vi "RingWithKerf.vi"(5 "Center Hole":dbl=1.0 format="%.2f", 6 "kerf?":bool, 7 "kerf space (cm)":dbl format="%.4f", 8 "Trans Geometry":T2={"Radius"=4.8, "a"=1.0, "focus location"=12.0} {"focus location" format="%.2f"; "a" format="%.2f"; "Radius" format="%.2f"}, 9 "Variables":T1={"Number of rings"=1, "sound spd (cm/s)"=150000, "z span (cm)"=4.0, "z steps"=20, "y spacing (cm)"=0.01, "y steps"=50, "time step (s)"=1e-08, "z"=0.0, "y"=0.0, "ref delay"=0.0, "freq (MHz)"=4.71, "cycles"=300} {"freq (MHz)" format="%.2f"; "z span (cm)" format="%.2f"; "y" format="%.2f"; "ref delay" format="%.2f"; "y spacing (cm)" format="%.2f"; "z" format="%.2f"; "time step (s)" format="%.2e"}) -> (0 "refdelay":dbl, 1 "appended array":cluster{"R":dbl, "a":dbl}[][](array[cluster]) {"a" format="%.2f"; "R" format="%.3f"})   [LabVIEW 2022 SP3]
panel:
  in  "Seno 30 mm R 18 mm Ap":cluster{"R":dbl, "a":dbl}[][](array[cluster])=[[{"R"=3.0, "a"=0.25145}, {"R"=0.0, "a"=0.0}], [{"R"=3.0, "a"=0.38285}, {"R"=3.0, "a"=0.28865}], [{"R"=3.0, "a"=0.4896}, {"R"=3.0, "a"=0.42005}], [{"R"=3.0, "a"=0.58375}, {"R"=3.0, "a"=0.5268}], [{"R"=3.0, "a"=0.66995}, {"R"=3.0, "a"=0.62095}], [{"R"=3.0, "a"=0.75055}, {"R"=3.0, "a"=0.70715}], [{"R"=3.0, "a"=0.8269}, {"R"=3.0, "a"=0.78775}], [{"R"=3.0, "a"=0.9}, {"R"=3.0, "a"=0.8641}]]
  in  "Seno 11 mm R 16 mm Ap":cluster{"R":dbl, "a":dbl}[][](array[cluster])=[[{"R"=1.1, "a"=0.2155}, {"R"=0.0, "a"=0.0}], [{"R"=1.1, "a"=0.3322}, {"R"=1.1, "a"=0.2527}], [{"R"=1.1, "a"=0.4277}, {"R"=1.1, "a"=0.3694}], [{"R"=1.1, "a"=0.5124}, {"R"=1.1, "a"=0.4649}], [{"R"=1.1, "a"=0.5904}, {"R"=1.1, "a"=0.5466}], [{"R"=1.1, "a"=0.6636}, {"R"=1.1, "a"=0.6261}], [{"R"=1.1, "a"=0.7332}, {"R"=1.1, "a"=0.7008}], [{"R"=1.1, "a"=0.7999101254524568}, {"R"=1.1, "a"=0.7704}]] {"a" format="%.4f"; "R" format="%.3f"}
  in  "Seno 25 mm R 16 mm App":cluster{"R":dbl, "a":dbl}[][](array[cluster])=[[{"R"=2.5, "a"=0.36477000000000004}, {"R"=0.0, "a"=0.0}], [{"R"=2.5, "a"=0.536}, {"R"=2.5, "a"=0.3972}], [{"R"=2.5, "a"=0.6769}, {"R"=2.5, "a"=0.5732}], [{"R"=2.5, "a"=0.799903752690246}, {"R"=2.5, "a"=0.7141}]] {"a" format="%.3f"; "R" format="%.3f"}
  out "Ring Areas cm^2":dbl[](array[numeric]) format="%.4f"
  # "5.029 \t0.000\n7.657 \t5.773\n9.792 \t8.401\n11.675 \t10.536\n13.399 \t12.419\n15.011 \t14.143\n16.538 \t15.755 \n18.000 \t17.282"
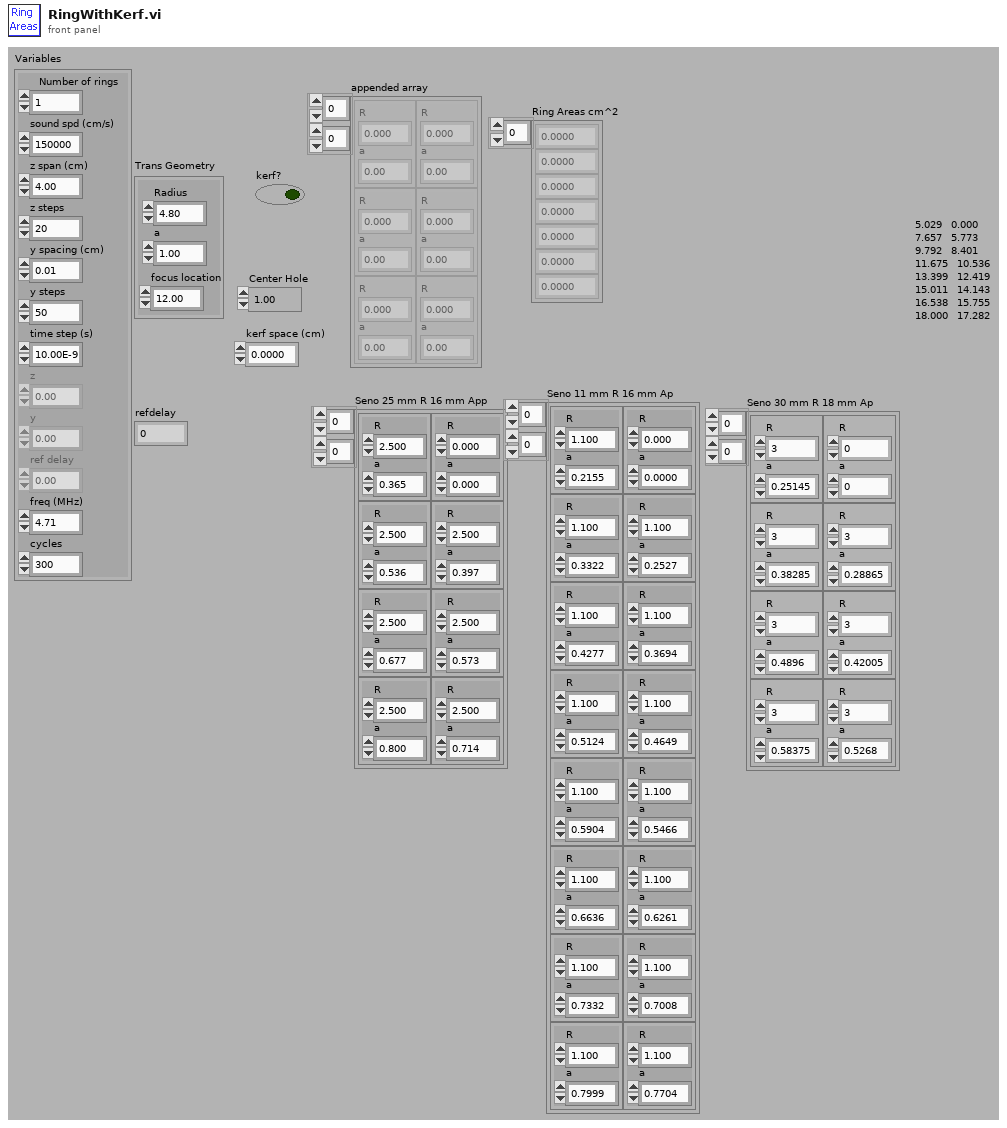
[diagram p1: front panel]
types:
  T1 = cluster{"Number of rings":i32, "sound spd (cm/s)":i32, "z span (cm)":dbl, "z steps":i32, "y spacing (cm)":dbl, "y steps":i32, "time step (s)":sgl, "z":dbl, "y":dbl, "ref delay":dbl, "freq (MHz)":dbl, "cycles":i32}
  T2 = cluster{"Radius":dbl, "a":dbl, "focus location":dbl}
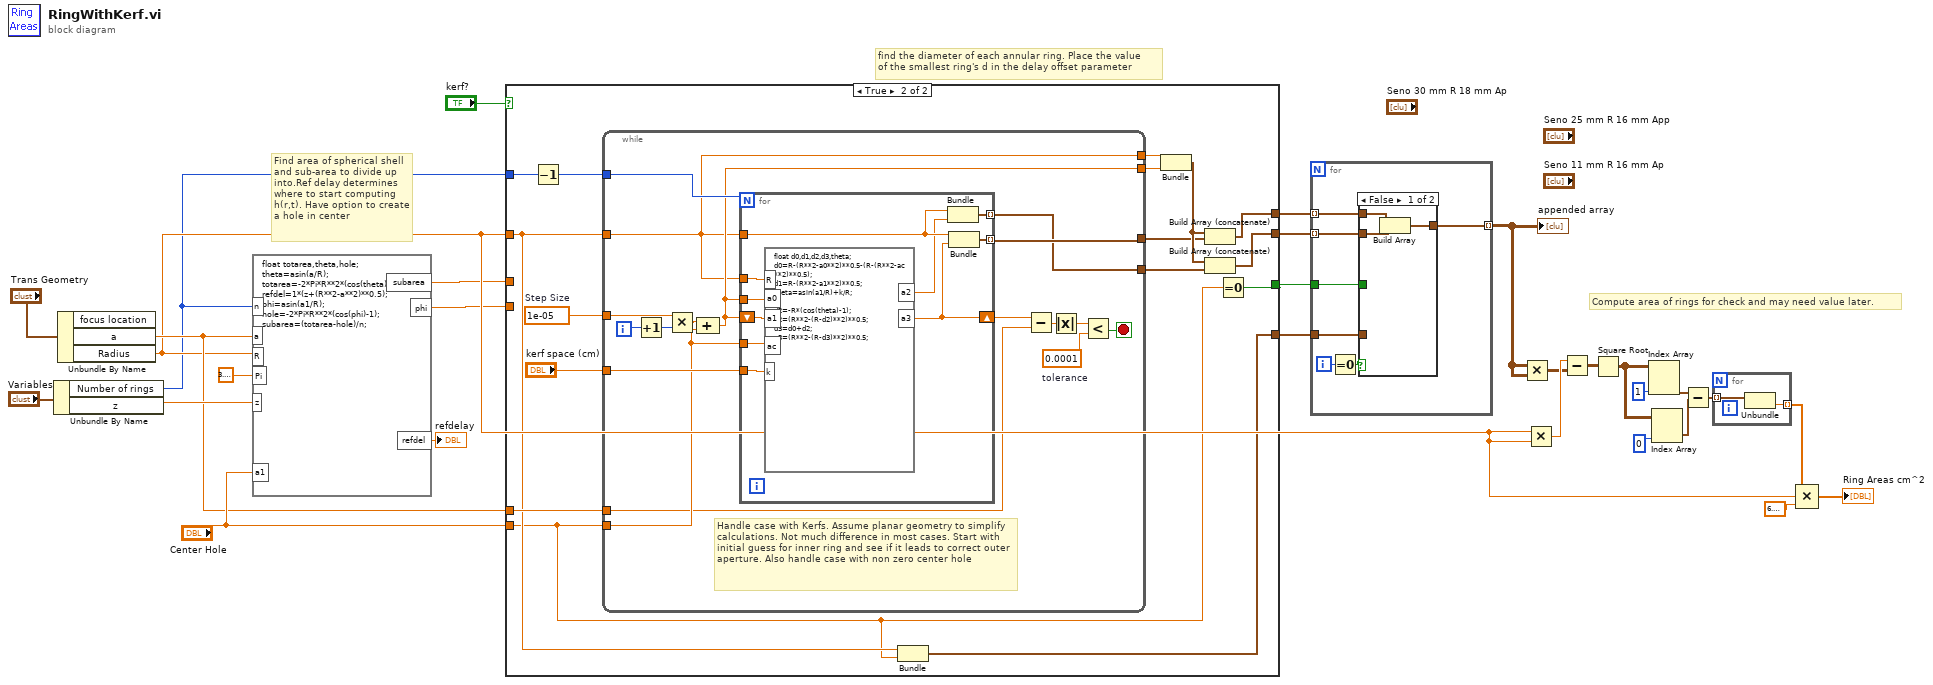
[diagram p0: block diagram]
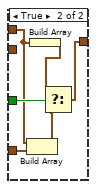
[diagram p2: hidden frame]
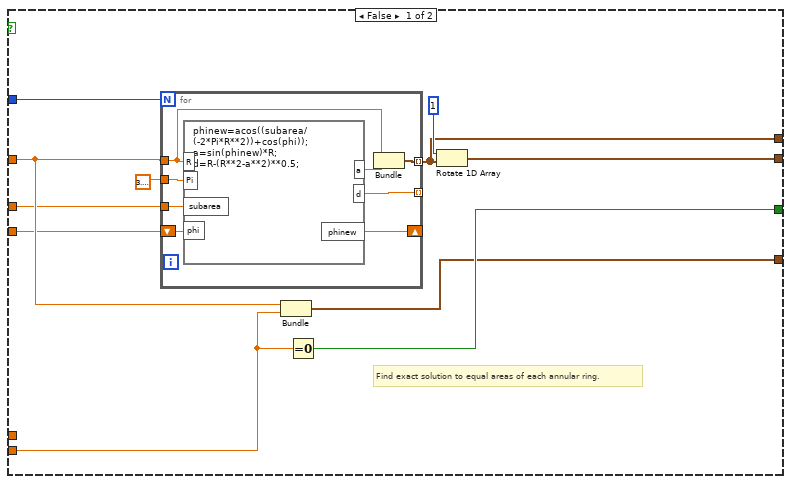
[diagram p3: hidden frame]
diagram:
  # "Find area of spherical shell and sub-area to divide up into.Ref delay determines where to start computing h(r,t). Have option to create a hole in center"
  # "Compute area of rings for check and may need value later."
  # "find the diameter of each annular ring. Place the value\nof the smallest ring's d in the delay offset parameter"
  n1 = Unbundle By Name("Variables") -> ("Number of rings"=w2:i32, "z"=w11:dbl)
  n2 = Unbundle By Name("Trans Geometry") -> ("a"=w8:dbl, "Radius"=w7:dbl)  [unwired: 1 out]
  n3 = formula code="float totarea,theta,hole;\ntheta=asin(a/R);\ntotarea=-2*Pi*R**2*(cos(theta)-1);\nrefdel=1*(z+(R**2-a**2)**0.5);\nphi=asin(a1/R);\nhole=-2*Pi*R**2*(cos(phi)-1);\nsubarea=(totarea-hole)/n;"("a"=w8, "R"=w7, "Pi"=3.141592653589793, "n"=w2, "z"=w11, "a1"="Center Hole") -> ("subarea"=w5:dbl, "refdel"=→"refdelay":dbl, "phi"=w6:dbl)
  n4 = case shown="True" "kerf?" {
    tunnel: w7 -> [w37 w50]
    tunnel: w8 -> [_ w63]
    tunnel: w2 -> [w38 w60]
    tunnel: "Center Hole" -> [w36 w49]
    tunnel: [w35 w54] -> w28
    tunnel: [w34 w53] -> w27
    tunnel: [w33 w52] -> w26
    tunnel: [w32 w51] -> w25
    tunnel: w6 -> [w31 _]
    tunnel: w5 -> [w30 _]
    frame False {
      # "Find exact solution to equal areas of each annular ring."
      n5 = for {
        N: w38 -> [_]
        tunnel: w30 -> [w48]
        tunnel: w37 -> [w41]
        tunnel: 3.141592653589793 -> [w47]
        shift-right: [w44] -> _
        shift-left: w31 -> [w46]
        tunnel: [w45] -> w35 mode=indexing
        tunnel: [w43] -> _ mode=indexing
        n6 = formula code="phinew=acos((subarea/(-2*Pi*R**2))+cos(phi));\na=sin(phinew)*R;\nd=R-(R**2-a**2)**0.5;"("subarea"=w48, "R"=w41, "Pi"=w47, "phi"=w46) -> ("phinew"=w44:dbl, "a"=w42:dbl, "d"=w43:dbl)
        n7 = Bundle("Radius"=w41, "a"=w42) -> (w45:cluster{"Radius":dbl, "a":dbl})  [unwired: 1 out]
      }
      n8 = Bundle("Radius"=w37, "Center Hole"=w36) -> (w32:cluster{"Radius":dbl, "Center Hole":dbl})  [unwired: 1 out]
      n9 = Equal To 0?(x=w36) -> (x = 0?=w33:bool)
      n10 = Rotate 1D Array(1:w35, 2:1) -> (0:w34:cluster{"Radius":dbl, "a":dbl}[])
    }
    frame True {
      w64 = 1e-05  # Step Size
      n11 = Decrement(x=w60) -> (x-1=w59:i32)
      n12 = while {
        tunnel: "kerf space (cm)" -> [w77]
        tunnel: w50 -> [w73]
        tunnel: [w78] -> w55
        tunnel: w64 -> [w79]
        tunnel: w63 -> [w69]
        tunnel: [w73] -> w62
        tunnel: [w74] -> w61
        tunnel: w59 -> [w76]
        tunnel: [w75] -> w56
        tunnel: w49 -> [w72]
        i -> [w81]
        stop <- w65 stop-if-true
        w66 = 0.0001  # tolerance
        # "Handle case with Kerfs. Assume planar geometry to simplify calculations. Not much difference in most cases. Start with initial guess for inner ring and see if it leads to correct outer aperture. Also handle case with non zero center hole"
        n13 = Increment(x=w81) -> (x+1=w71:i32)
        n14 = Multiply(x=w79, y=w71) -> (x*y=w80:dbl)
        n15 = Compound Arithmetic op=ADD(w80, w72) -> (w74:dbl)
        n16 = for {
          N: w76 -> [_]
          tunnel: w77 -> [w86]
          shift-right: [w83] -> w70
          shift-left: w74 -> [w87]
          tunnel: w73 -> [w90]
          tunnel: [w91] -> w78 mode=indexing
          tunnel: [w89] -> w75 mode=indexing
          tunnel: w74 -> [w88]
          tunnel: w73 -> [w85]
          tunnel: w72 -> [w82]
          n17 = formula code="float d0,d1,d2,d3,theta;\nd0=R-(R**2-a0**2)**0.5-(R-(R**2-ac**2)**0.5);\nd1=R-(R**2-a1**2)**0.5;\ntheta=asin(a1/R)+k/R;\n\nd2=-R*(cos(theta)-1);\na2=(R**2-(R-d2)**2)**0.5;\nd3=d0+d2;\na3=(R**2-(R-d3)**2)**0.5;"("k"=w86, "a0"=w88, "R"=w85, "a1"=w87, "ac"=w82) -> ("a3"=w83:dbl, "a2"=w84:dbl)
          n18 = Bundle("Radius"=w90, "a2"=w84) -> (w89:cluster{"Radius":dbl, "a2":dbl})  [unwired: 1 out]
          n19 = Bundle("Radius"=w90, "a3"=w83) -> (w91:cluster{"Radius":dbl, "a3":dbl})  [unwired: 1 out]
        }
        n20 = Subtract(x=w70, y=w69) -> (x-y=w68:dbl)
        n21 = Absolute Value(x=w68) -> (abs(x)=w67:dbl)
        n22 = Less?(x=w67, y=w66) -> (x < y?=w65:bool)
      }
      n23 = Bundle("Radius"=w50, "Center Hole"=w49) -> (w51:cluster{"Radius":dbl, "Center Hole":dbl})  [unwired: 1 out]
      n24 = Bundle("Radius"=w62, w61) -> (w58:cluster{"Radius":dbl, dbl})  [unwired: 1 out]
      n25 = Build Array (concatenate)(w58, w55) -> (w54:cluster{"Radius":dbl, "a3":dbl}[])
      n26 = Build Array (concatenate)(w58, w56) -> (w53:cluster{"Radius":dbl, "a2":dbl}[])
      n27 = Equal To 0?(x=w49) -> (x = 0?=w52:bool)
    }
  }
  n28 = for {
    tunnel: w28 -> [w98] mode=indexing
    tunnel: w27 -> [w97] mode=indexing
    tunnel: w25 -> [w94]
    tunnel: w26 -> [w93]
    tunnel: [w92] -> w1 mode=indexing
    i -> [w96]
    n29 = Equal To 0?(x=w96) -> (x = 0?=w95:bool)
    n30 = case shown="False" w95 {
      tunnel: [w101 w104] -> w92
      tunnel: w97 -> [w99 _]
      tunnel: w98 -> [w100 w102]
      tunnel: w93 -> [_ w106]
      tunnel: w94 -> [_ w103]
      frame False {
        n31 = Build Array(w100, w99) -> (w101:cluster{"Radius":dbl, "a2":dbl}[])
      }
      frame True {
        n32 = Build Array(w102, w103) -> (w105:cluster{"Radius":dbl, "Center Hole":dbl}[])
        n33 = Build Array(w102) -> (w107:cluster{"Radius":dbl, "a3":dbl}[])
        n34 = Select(t=w107, s=w106, f=w105) -> (s? t:f=w104:cluster{"Radius":dbl, "Center Hole":dbl}[])
      }
    }
  }
  "appended array" <- w1
  n35 = Multiply(x=w1, y=w1) -> (x*y=w23:cluster{"Radius":dbl, "Center Hole":dbl}[][])
  n36 = Multiply(x=w7, y=w7) -> (x*y=w24:dbl)
  n37 = Subtract(x=w24, y=w23) -> (x-y=w22:cluster{"Radius":dbl, "Center Hole":dbl}[][])
  n38 = Square Root(x=w22) -> (sqrt(x)=w21:cluster{"Radius":dbl, "Center Hole":dbl}[][])
  n39 = Index Array(array=w21, index (col)=1) -> (element=w20:cluster{"Radius":dbl, "Center Hole":dbl}[])  [unwired: 1 in]
  n40 = Index Array(array=w21, index (col)=0) -> (element=w19:cluster{"Radius":dbl, "Center Hole":dbl}[])  [unwired: 1 in]
  n41 = Subtract(x=w20, y=w19) -> (x-y=w18:cluster{"Radius":dbl, "Center Hole":dbl}[])
  n42 = for {
    tunnel: w18 -> [w109] mode=indexing
    tunnel: [w108] -> w14 mode=indexing
    n43 = Unbundle(w109) -> ("Center Hole"=w108:dbl)  [unwired: 1 out]
  }
  n44 = Compound Arithmetic op=MULTIPLY(w14, w7, 6.283185307179586) -> (→"Ring Areas cm^2":dbl[])
